vi "E441X_PM_Reset.vi"(0 "VISA session":refnum<visa-resource-name>, 11 "error in (no error)":errorcluster {"code" format="%.0x"}) -> (4 "dup VISA session":refnum<visa-resource-name>, 15 "error out":errorcluster {"code" format="%.0x"})   [LabVIEW 2015]
doc: "This VI resets the instrument, and then sends a set of default setup commands to the instrument."
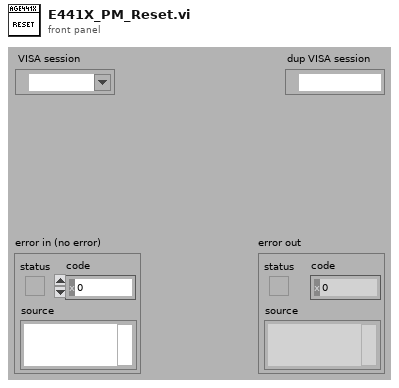
[diagram p1: front panel]
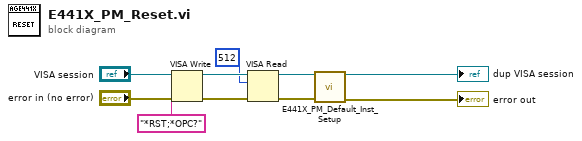
[diagram p0: block diagram]
diagram:
  n1 = VISA Write(VISA resource name="VISA session", write buffer="*RST;*OPC?" ("Reset Command"), error in (no error)="error in (no error)") -> (VISA resource name out=w5:refnum<visa-resource-name>, error out=w4:errorcluster)  [unwired: 1 out]
  n2 = VISA Read(VISA resource name=w5, byte count=u32 512 ("byte count (0)"), error in (no error)=w4) -> (VISA resource name out=w2:refnum<visa-resource-name>, error out=w3:errorcluster)  [unwired: 2 out]
  n3 = call "E441X_PM_Default_Inst_Setup.vi"("VISA session"=w2, "error in (no error)"=w3) -> ("dup VISA session"=→"dup VISA session":refnum<visa-resource-name>, "error out"=→"error out":errorcluster)  [unwired: 12 in]
